vi "subGetLibraryDependencies.vi"(8 "error in (no error)":errorcluster, 11 "Project ref":refnum<vi>) -> (0 "error out":errorcluster, 1 "Library refs":map{string, refnum<vi>}(c390), 3 "Deps":map{string, set{string}}(c390))   [LabVIEW 2020, in "SolutionBuilder.lvlib"]
uses:
  SolutionBuilder.lvlib
  <vilib>/Utility/miscctls.llb/LVMapReplaceAction.ctl
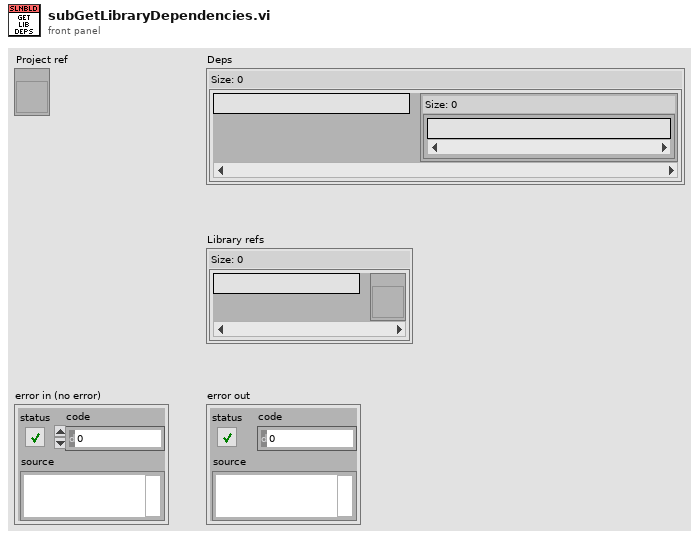
[diagram p1: front panel]
types:
  T1 = typedef "LVMapReplaceAction.ctl" = enum32{"Modify Entry only if found", "Add or Modify Entry", "Delete Entry"}
  T2 = typedef "NI_FileType.lvlib/LVFileType.ctl" = enum32{"Invalid file", "Unknown type", "Instrument", "Control", "Polymorphic VI", "Project", "Library", "LVClass", "XControl", "XNode", "Shared library", ".NET assembly", "ActiveX interface", "CIN", "Run-time menu", "Palette menu", "Help file", "LLB", "XNode Edit Dependency", "Class Private Data Control", "Statechart", "MathScript .m file", "Ladder Diagram", "LVLibp", "XNode Build Dependency"}
  T3 = cluster{"path":path, "delimited name":string, "type":T2, "iState":u32, "iStyle":u16, "wStyle":u16, "buttons":u16, "viflags":u32, "viflags2":u32, "links":u32[]}[]
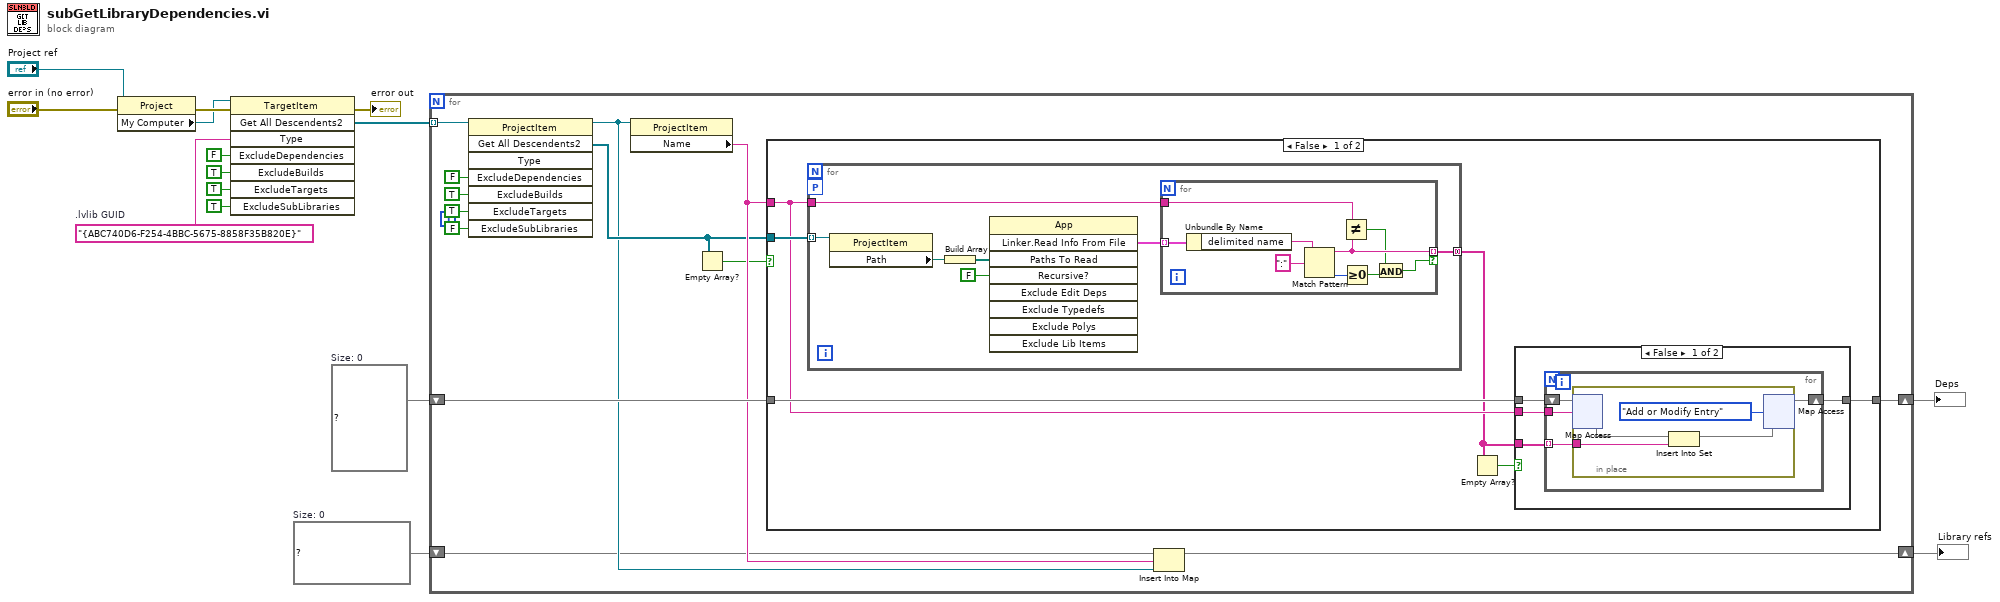
[diagram p0: block diagram]
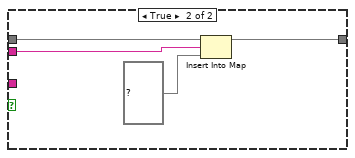
[diagram p2: hidden frame]
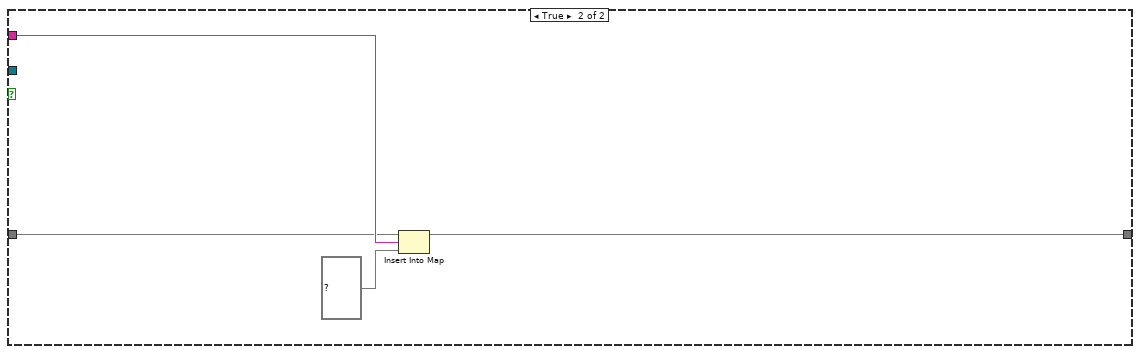
[diagram p3: hidden frame]
diagram:
  w2 = map{string, refnum<vi>} {}  # Size: 0
  w12 = map{string, set{string}} {}  # Size: 0
  w10 = "{ABC740D6-F254-4BBC-5675-8858F35B820E}"  # .lvlib GUID
  n1 = property class="Project"(reference="Project ref", error in="error in (no error)") -> (error out=w14:errorcluster, "My Computer"=w13:refnum<vi>)  [unwired: 1 out]
  n2 = invoke class="TargetItem" method="Get All Descendents2"(reference=w13, error in=w14, "Type"=w10, "ExcludeDependencies"=FALSE, "ExcludeBuilds"=TRUE, "ExcludeTargets"=TRUE, "ExcludeSubLibraries"=TRUE) -> (error out=→"error out":errorcluster, "Get All Descendents2"=w15:refnum<vi>[])  [unwired: 1 in, 6 out]
  n3 = for {
    tunnel: w15 -> [w26] mode=indexing
    shift-right: [w27] -> w11
    shift-left: w12 -> [w28]
    shift-right: [w17] -> w1
    shift-left: w2 -> [w16]
    n4 = invoke class="ProjectItem" method="Get All Descendents2"(reference=w26, "ExcludeDependencies"=FALSE, "ExcludeBuilds"=TRUE, "ExcludeTargets"=TRUE, "ExcludeSubLibraries"=FALSE) -> (reference out=w18:refnum<vi>, "Get All Descendents2"=w24:refnum<vi>[])  [unwired: 3 in, 6 out]
    n5 = property class="ProjectItem"(reference=w18) -> ("Name"=w25:string)  [unwired: 1 in, 2 out]
    n6 = Empty Array?(array=w24) -> (empty?=w23:bool)
    n7 = case shown="False" w23 {
      tunnel: w28 -> [w34 w69]
      tunnel: [w33 w68] -> w27
      tunnel: w24 -> [w32 _]
      tunnel: w25 -> [w31 w70]
      frame False {
        n8 = for {
          tunnel: w32 -> [w57] mode=indexing
          workers-P: _ -> [_]
          tunnel: [w52] -> w30 mode=concatenating
          tunnel: w31 -> [w51]
          n9 = property class="ProjectItem"(reference=w57) -> ("Path"=w55:path)  [unwired: 1 in, 2 out]
          n10 = Build Array(w55) -> (w54:path[])
          n11 = invoke class="App" method="Linker.Read Info From File"("Paths To Read"=w54, "Recursive?"=FALSE) -> ("Linker.Read Info From File"=w53:T3)  [unwired: 7 in, 8 out]
          n12 = for {
            tunnel: w53 -> [w66] mode=indexing
            tunnel: [w61] -> w52 mode=indexing if=w58
            tunnel: w51 -> [w62]
            n13 = Unbundle By Name(w66) -> ("delimited name"=w64:string)
            n14 = Match Pattern(string=w64, regular expression=":") -> (before substring=w61:string, offset past match=w63:i32)  [unwired: 1 in, 2 out]
            n15 = Not Equal?(x=w62, y=w61) -> (x != y?=w60:bool)
            n16 = Greater Or Equal To 0?(x=w63) -> (x >= 0?=w59:bool)
            n17 = And(x=w60, y=w59) -> (x .and. y?=w58:bool)
          }
        }
        n18 = Empty Array?(array=w30) -> (empty?=w29:bool)
        n19 = case shown="False" w29 {
          tunnel: w34 -> [w38 w49]
          tunnel: [w37 w48] -> w33
          tunnel: w31 -> [w36 w47]
          tunnel: w30 -> [w35 _]
          frame False {
            n20 = for {
              shift-right: [w41] -> w37
              shift-left: w38 -> [w42]
              tunnel: w36 -> [w40]
              tunnel: w35 -> [w39] mode=indexing
              n21 = in-place {
                in-place-border: w39 -> [w45]
                n22 = in-place-map #1(w42, w40) -> (w46:set{string})  [unwired: 1 in, 1 out]
                n23 = Insert Into Set(10:w45, 11:w46) -> (3:w44:set{string})  [unwired: 1 out]
                n24 = in-place-map #1(w44, LVMapReplaceAction."Add or Modify Entry" ("action")) -> (w41:map{string, set{string}})  [unwired: 2 out]
              }
            }
          }
          frame True {
            n25 = Insert Into Map(map in=w49, key=w47, value=set{string} {}) -> (map out=w48:map{string, set{string}})  [unwired: 2 out]
          }
        }
      }
      frame True {
        n26 = Insert Into Map(map in=w69, key=w70, value=set{string} {}) -> (map out=w68:map{string, set{string}})  [unwired: 2 out]
      }
    }
    n27 = Insert Into Map(map in=w16, key=w25, value=w18) -> (map out=w17:map{string, refnum<vi>})  [unwired: 2 out]
  }
  "Deps" <- w11
  "Library refs" <- w1
